vi "Edge Detection with 2D Convolution.vi"() -> ()   [LabVIEW 2011]
doc: "This VI uses two-dimensional convolution to perform image edge detection.\n\nNote: You can use this example only in the LabVIEW Full or Professional Development Systems."
uses:
  <vilib>/Analysis/Matrix/Datatypes/RealMatrix.ctl
  <vilib>/Analysis/2dsp.llb/2D Convolution (DBL).vi
  <vilib>/Analysis/NI_AALPro.lvlib
  <vilib>/Analysis/Matrix/NI_Matrix.lvlib
panel:
  in  "File Path":path=path "X:/Cloud Drives/Dropbox/Europhotonics/FringeMan/Image Storage/Unwrapped Phase Maps/5 Fringes/strong_dist.png"
  in  "Operator selection":enum16{"Laplacian Type I", "Laplacian Type II"}(ring)
  in  "stop":bool
  out "Edge Image":dbl[][](graph)
  out "Convolution operator":T1=[[1.0, 1.0, 1.0], [1.0, -8.0, 1.0], [1.0, 1.0, 1.0]]
  out "Source Image":u8[][](graph)
  # "2D Convolution for Image Edge Detection"
  # "Select Help»Show Context Help and move the cursor over the VI icon to display help for this VI.\n\nInstructions: \n1) Run the VI\n2) Change between images and Operators to see the difference in the Edge Image\n3) Look at the block diagram for more information"
  # "Convolution"
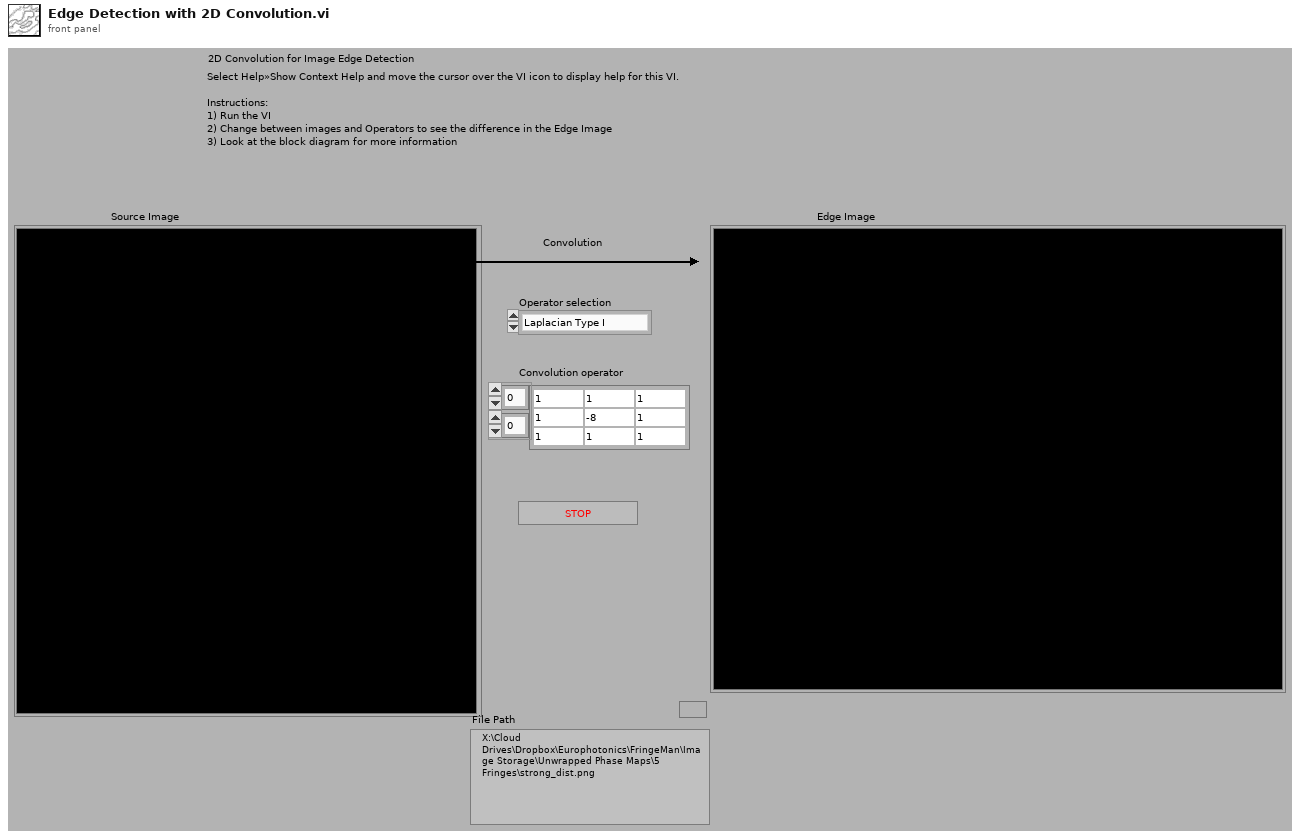
[diagram p1: front panel]
types:
  T1 = typedef "NI_Matrix.lvlib/RealMatrix.ctl" = dbl[][]
  T2 = typedef "IMAQ Image.ctl" = refnum<image>
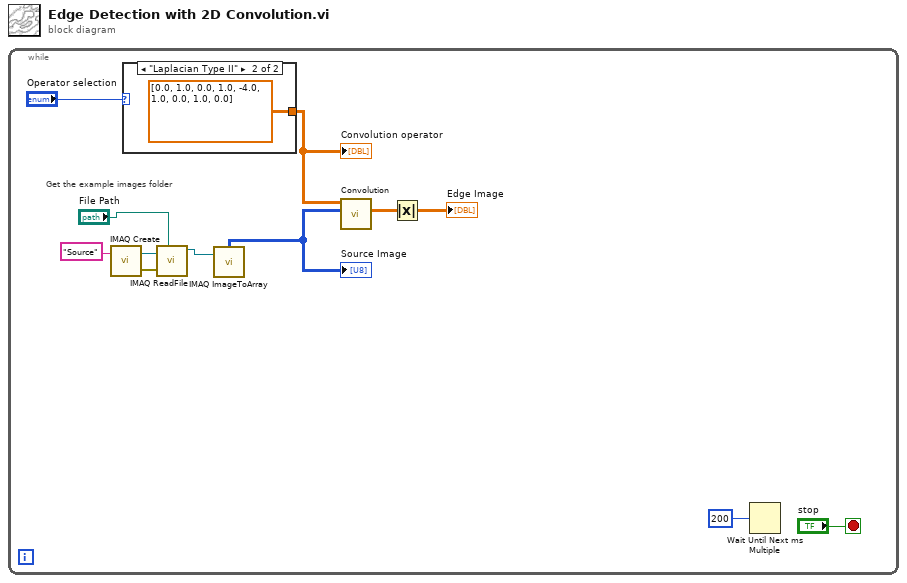
[diagram p0: block diagram]
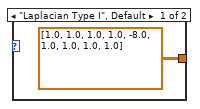
[diagram p2: hidden frame]
diagram:
  n1 = while {
    stop <- "stop" stop-if-true
    # "Get the example images folder"
    n2 = call "IMAQ Create"("Image Name"="Source") -> ("New Image"=w5:T2, "error out"=w4:errorcluster)  [unwired: 3 in, 1 out]
    n3 = case shown="\"Laplacian Type II\"" "Operator selection" {
      tunnel: [dbl[][] [[1.0, 1.0, 1.0], [1.0, -8.0, 1.0], [1.0, 1.0, 1.0]] dbl[][] [[0.0, 1.0, 0.0], [1.0, -4.0, 1.0], [0.0, 1.0, 0.0]]] -> w7
      frame "Laplacian Type I", Default {
      }
      frame "Laplacian Type II" {
      }
    }
    "Convolution operator" <- w7
    n4 = call "IMAQ ReadFile"("File Path"="File Path", "error in (no error)"=w4, "Image"=w5) -> ("Image Out"=w2:T2)  [unwired: 2 in, 6 out]
    n5 = call "IMAQ ImageToArray"("Image"=w2) -> ("Image Pixels (U8)"=w1:u8[][])  [unwired: 3 in, 4 out]
    "Source Image" <- w1
    n6 = call-poly <vilib>:"Convolution.vi"("Y"=w1, "X"=w7) -> ("X * Y"=w12:dbl[][])  [unwired: 8 in, 1 out]
    n7 = Absolute Value(x=w12) -> (abs(x)=→"Edge Image":dbl[][])
    n8 = Wait Until Next ms Multiple(millisecond multiple=u32 200) -> ()  [unwired: 1 out]
  }
